vi "LPCA Interface Front Panel Update (Sub-Vi).vi"(6 "byte count":u32, 7 "String":refnum<vi>, 8 "error in (no error)":errorcluster, 9 "regular expression":string, 10 "VISA resource name":refnum<visa-resource-name>, 11 "Cluster":T1={"Queue Array"=[], "Queue Element"={"state"="", "data"=variant}, "System Event"=refnum, "System Event RefNum"=refnum, "Queue List"=[], "LPCA COM"="", "Rotating"=FALSE, "PrecorAI"="", "T_0 Index"=0, "Bar Graph X"=[], "Channels"=[], "Active Indicies"=[], "Active Channels"=[], "Sample Frequency"=0.0, "Ibrake Sweep"=[], "RPM Sweep"=[], "Load Sweep"=[], "Step Height Sweep"=[], "Range Sweep"=[], "A Counter"=0, "B Counter"=0, "C Counter"=0, "#A"=0, "#B"=0, "#C"=0, "Current RPM"=0.0, "Current Ibrake"=0, "Current Range"=0, "Current Step Height"=0, "Load Bank"=enum."OFF", "Cfg Cntrls"=[], "T_Monitor Indices"=[], "Thermal Limit"=0, "Thermal Resume"=0, "Timer Reset"=FALSE, "Stop Time"=0.0, "Autotest"=FALSE, "Pulsed RPM Capture"=FALSE, "Get Sample"=FALSE, "Last State"="", "Reset Timeout"=FALSE, "Ctrl Refs"={"Test Details"=refnum, "Save Config"=refnum, "Load Config"=refnum, "Path"=refnum, "Snapshot"=refnum, "SS#"=refnum, "Ibrake"=refnum, "RPM Target"=refnum, "Spin"=refnum, "Load Bank"=refnum, "Start Test"=refnum, "Pause Test"=refnum, "Load Sweep"=refnum, "RPM Sweep"=refnum, "Ibrake Sweep"=refnum, "Filters"=refnum, "Sample Frequency"=refnum, "Data Setup"=refnum, "Pause"=refnum, "Stop Time"=refnum, "S Period"=refnum, "Range"=refnum, "Step Height"=refnum, "Step Height Sweep"=refnum, "Range Sweep"=refnum, "Available Tests"=refnum, "RPM Graph"=refnum, "RPM Knob"=refnum, "FanMode"=refnum, "Fan Mode LED Array"=refnum, "Thermal Equilibrium"=refnum, "Data Display"=refnum, "LPCA Error"=refnum, "LPCA Ramp"=refnum, "LPCA Range"=refnum, "LPCA Resistance"=refnum, "Analyze Read"=refnum, "Console Select"=refnum, "Sub Panel"=refnum}, "Pulse Waveform"={"t0"=timestamp(0 s since 1904-01-01), "dt"=1.0, "Y"=[]}, "Snapshot"={"Test Details"="test", "Version"="test", "Date"=timestamp(3493915594.3018084 s since 1904-01-01), "Selected Test"="man", "Snapshot Number"=0, "Time"=timestamp(3493915602.7292905 s since 1904-01-01), "Ibrake Setpoint"="1", "RPM Setpoint"="20", "Range Setpoint"="", "Step Height Setpoint"="", "Load Bank Setpoint"="15", "Measurement Headers"="a,b,c,1,2,3", "Measurements"="1,2,3,4,5,6,7,8", "A"=0, "B"=0, "C"=0, "Raw Data"=[], "Available Tests"=enum."Manual", "Ibrake List"="", "RPM List"="", "Load Bank List"="", "Range List"="", "Step Height List"="", "FanMode Setpoint"=enum."Auto"}, "Sample Period"=0.0, "OverTemp"=FALSE, "Available Tests"=enum."Manual", "FanMode"=enum."Auto", "Fan Mode LED Array"=[FALSE, TRUE, FALSE], "Thermal\nEquilibrium "=FALSE, "Equilibrium Stop"=FALSE, "AvgDegChg"=[]} {"Snapshot"."Time" format="%<%H:%M:%S>T"; "Snapshot"."Date" format="%<%m/%d/%Y>T"}) -> (0 "error out":errorcluster, 3 "VISA resource out":refnum<visa-resource-name>)   [LabVIEW 2017]
uses:
  Controls/Test TypeDef.ctl
  Code Library/Queue References Array.ctl
  Code Library/Queue Element.ctl
  Controls/Load Bank.ctl
  Controls/Available Tests.ctl
  Console Sim/Controls/Console Select.ctl
  Controls/Snapshot Typedef.ctl
  Controls/FanMode.ctl
  <vilib>/regexp/Match Regular Expression.xnode
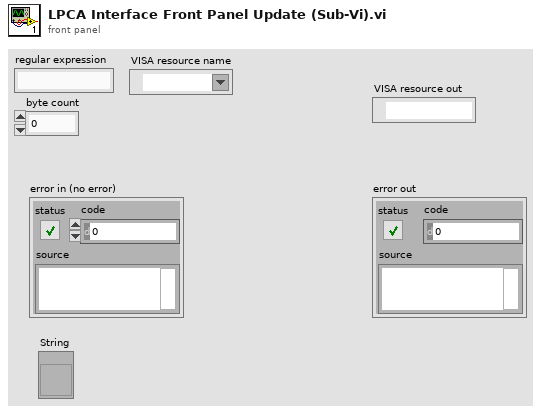
[diagram p1: front panel]
types:
  T1 = typedef "Test TypeDef.ctl" = cluster{"Queue Array":T2, "Queue Element":T3, "System Event":refnum<user-event>, "System Event RefNum":refnum<event-registration>, "Queue List":string[], "LPCA COM":refnum<visa-resource-name>, "Rotating":bool, "PrecorAI":refnum<k21>, "T_0 Index":i32, "Bar Graph X":i32[], "Channels":string[], "Active Indicies":i32[], "Active Channels":string[][], "Sample Frequency":dbl, "Ibrake Sweep":string[], "RPM Sweep":string[], "Load Sweep":string[], "Step Height Sweep":string[], "Range Sweep":string[], "A Counter":i32, "B Counter":i32, "C Counter":i32, "#A":i32, "#B":i32, "#C":i32, "Current RPM":dbl, "Current Ibrake":u32, "Current Range":u32, "Current Step Height":u32, "Load Bank":T4, "Cfg Cntrls":refnum<vi>[], "T_Monitor Indices":i32[], "Thermal Limit":i32, "Thermal Resume":i32, "Timer Reset":bool, "Stop Time":dbl, "Autotest":bool, "Pulsed RPM Capture":bool, "Get Sample":bool, "Last State":string, "Reset Timeout":bool, "Ctrl Refs":cluster{"Test Details":refnum<vi>, "Save Config":refnum<vi>, "Load Config":refnum<vi>, "Path":refnum<vi>, "Snapshot":refnum<vi>, "SS#":refnum<vi>, "Ibrake":refnum<vi>, "RPM Target":refnum<vi>, "Spin":refnum<vi>, "Load Bank":refnum<vi>, "Start Test":refnum<vi>, "Pause Test":refnum<vi>, "Load Sweep":refnum<vi>, "RPM Sweep":refnum<vi>, "Ibrake Sweep":refnum<vi>, "Filters":refnum<vi>, "Sample Frequency":refnum<vi>, "Data Setup":refnum<vi>, "Pause":refnum<vi>, "Stop Time":refnum<vi>, "S Period":refnum<vi>, "Range":refnum<vi>, "Step Height":refnum<vi>, "Step Height Sweep":refnum<vi>, "Range Sweep":refnum<vi>, "Available Tests":refnum<vi>, "RPM Graph":refnum<vi>, "RPM Knob":refnum<vi>, "FanMode":refnum<vi>, "Fan Mode LED Array":refnum<vi>, "Thermal Equilibrium":refnum<vi>, "Data Display":refnum<vi>, "LPCA Error":refnum<vi>, "LPCA Ramp":refnum<vi>, "LPCA Range":refnum<vi>, "LPCA Resistance":refnum<vi>, "Analyze Read":refnum<vi>, "Console Select":refnum<vi>, "Sub Panel":refnum<vi>}, "Pulse Waveform":waveform(dbl), "Snapshot":T5, "Sample Period":dbl, "OverTemp":bool, "Available Tests":T6, "FanMode":T7, "Fan Mode LED Array":bool[], "Thermal\nEquilibrium ":bool, "Equilibrium Stop":bool, "AvgDegChg":dbl[]}
  T2 = typedef "Queue References Array.ctl" = refnum<queue>[]
  T3 = typedef "Queue Element.ctl" = cluster{"state":string, "data":variant}
  T4 = typedef "Load Bank.ctl" = enum16{"OFF", "50", "25", "16.7", "12.5", "10.0", "8.3", "7.1", "6.3", "5.6", "5.0", "4.5", "4.2", "3.8", "3.6", "3.3", "3.1"}
  T5 = typedef "Snapshot Typedef.ctl" = cluster{"Test Details":string, "Version":string, "Date":timestamp, "Selected Test":string, "Snapshot Number":u16, "Time":timestamp, "Ibrake Setpoint":string, "RPM Setpoint":string, "Range Setpoint":string, "Step Height Setpoint":string, "Load Bank Setpoint":string, "Measurement Headers":string, "Measurements":string, "A":i32, "B":i32, "C":i32, "Raw Data":string[][], "Available Tests":T6, "Ibrake List":string, "RPM List":string, "Load Bank List":string, "Range List":string, "Step Height List":string, "FanMode Setpoint":T7}
  T6 = typedef "Available Tests.ctl" = enum16{"Manual", "EFX Brake Torque", "Generator Torque", "EFX Brake Thermal", "Generator Thermal", "Pulsed RPM", "AMT Brake Torque", "Bike Brake Torque", "AMT Brake Thermal", "Bike Brake Thermal"}
  T7 = typedef "FanMode.ctl" = enum16{"On", "Off", "Auto"}
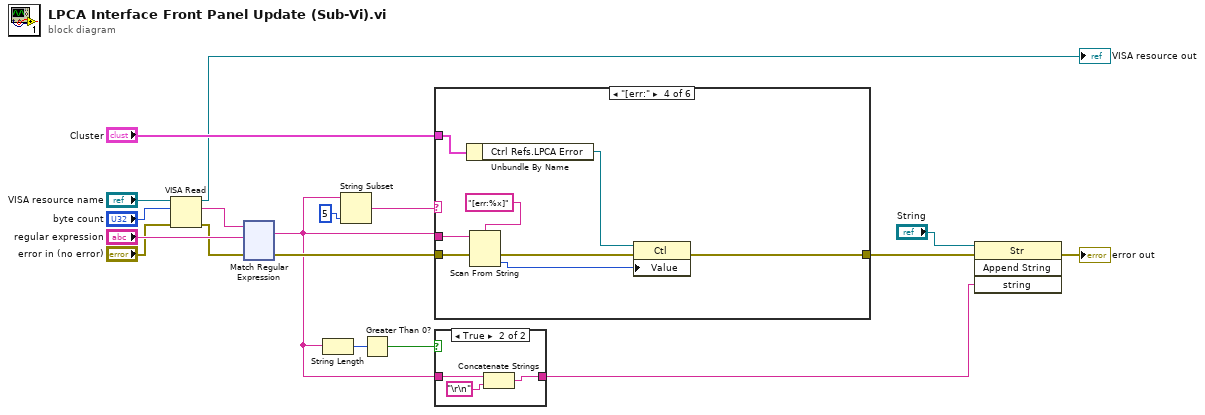
[diagram p0: block diagram]
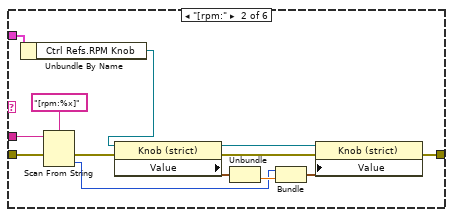
[diagram p4: hidden frame]
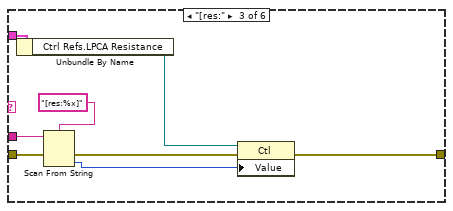
[diagram p5: hidden frame]
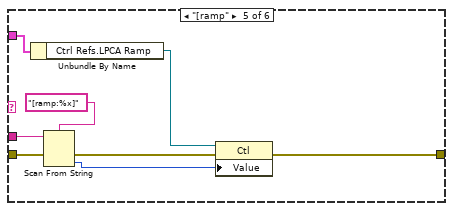
[diagram p6: hidden frame]
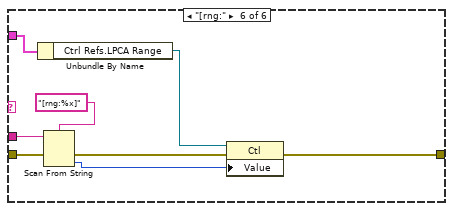
[diagram p7: hidden frame]
diagram:
  n1 = VISA Read(VISA resource name="VISA resource name", byte count="byte count", error in (no error)="error in (no error)") -> (VISA resource name out=→"VISA resource out":refnum<visa-resource-name>, read buffer=w6:string, error out=w7:errorcluster)  [unwired: 1 out]
  n2 = xnode "Match Regular Expression"("input string"=w6, "regular expression"="regular expression", "error in"=w7) -> ("whole match"=w3:string, "error out"=w11:errorcluster)  [unwired: 3 in, 3 out]
  n3 = String Length(string=w3) -> (length=w5:i32)
  n4 = String Subset(string=w3, length (rest)=5 ("length (rest)")) -> (substring=w18:string)  [unwired: 1 in]
  n5 = Greater Than 0?(x=w5) -> (x > 0?=w4:bool)
  n6 = case shown="\"[err:\"" w18 {
    tunnel: w11 -> [w19 w31 w39 w47 w55 w63]
    tunnel: [w19 w23 w33 w44 w52 w60] -> w14
    tunnel: w3 -> [_ w22 w37 w45 w53 w61]
    tunnel: "Cluster" -> [_ w21 w36 w42 w50 w58]
    frame "False", Default {
    }
    frame "[rpm:" {
      n7 = Unbundle By Name(w21) -> ("Ctrl Refs.RPM Knob"=w20:refnum<vi>)
      n8 = Scan From String(format string="[rpm:%x]", input string=w22, error in=w31) -> (error out=w25:errorcluster, output 1=w24:u32)  [unwired: 2 in, 2 out]
      n9 = property class="Knob (strict)"(reference=w20, error in=w25) -> (reference out=w29:refnum<vi>, error out=w30:errorcluster, "Value"=w26:cluster{dbl, dbl})
      n10 = Unbundle(w26) -> (w27:dbl)  [unwired: 1 out]
      n11 = Bundle(w24, w27) -> (w28:cluster{u32, dbl})  [unwired: 1 in]
      n12 = property class="Knob (strict)"(reference=w29, error in=w30, "Value"=w28) -> (error out=w23:errorcluster)  [unwired: 1 out]
    }
    frame "[res:" {
      n13 = Unbundle By Name(w36) -> ("Ctrl Refs.LPCA Resistance"=w34:refnum<vi>)
      n14 = Scan From String(format string="[res:%x]", input string=w37, error in=w39) -> (error out=w38:errorcluster, output 1=w35:u32)  [unwired: 2 in, 2 out]
      n15 = property class="Ctl"(reference=w34, error in=w38, "Value"=w35) -> (error out=w33:errorcluster)  [unwired: 1 out]
    }
    frame "[err:" {
      n16 = Unbundle By Name(w42) -> ("Ctrl Refs.LPCA Error"=w41:refnum<vi>)
      n17 = Scan From String(format string="[err:%x]", input string=w45, error in=w47) -> (error out=w46:errorcluster, output 1=w43:u32)  [unwired: 2 in, 2 out]
      n18 = property class="Ctl"(reference=w41, error in=w46, "Value"=w43) -> (error out=w44:errorcluster)  [unwired: 1 out]
    }
    frame "[ramp" {
      n19 = Unbundle By Name(w50) -> ("Ctrl Refs.LPCA Ramp"=w49:refnum<vi>)
      n20 = Scan From String(format string="[ramp:%x]", input string=w53, error in=w55) -> (error out=w54:errorcluster, output 1=w51:u32)  [unwired: 2 in, 2 out]
      n21 = property class="Ctl"(reference=w49, error in=w54, "Value"=w51) -> (error out=w52:errorcluster)  [unwired: 1 out]
    }
    frame "[rng:" {
      n22 = Unbundle By Name(w58) -> ("Ctrl Refs.LPCA Range"=w57:refnum<vi>)
      n23 = Scan From String(format string="[rng:%x]", input string=w61, error in=w63) -> (error out=w62:errorcluster, output 1=w59:u32)  [unwired: 2 in, 2 out]
      n24 = property class="Ctl"(reference=w57, error in=w62, "Value"=w59) -> (error out=w60:errorcluster)  [unwired: 1 out]
    }
  }
  n25 = case shown="True" w4 {
    tunnel: w3 -> [w65 w66]
    tunnel: [w65 w67] -> w2
    frame False {
    }
    frame True {
      n26 = Concatenate Strings(w66, "\r\n") -> (w67:string)
    }
  }
  n27 = invoke on="Invoke Node" class="Str" method="Append String"(reference="String", error in=w14, "string"=w2) -> (error out=→"error out":errorcluster)  [unwired: 1 in, 3 out]
